vi "RRTAsynCall.vi"(8 "error in (no error)":errorcluster, 9 "appended path":path, 10 "VI Refnum":refnum<vi>, 11 "Input":T1={"seed"=500000, "pathsize"=0, "probGoal"=0.1, "probWaypoint"=0.6, "step"=10.0, "threshold"=10.0, "field_length"=9000.0, "field_width"=6000.0, "startAndEnd"=[[0.0, 0.0], [0.0, 0.0]], "obsList"=[[0.0, 0.0]], "obsLen"=1, "lastTree"=[[0.0, 0.0]], "lastTreeLen"=1, "newTree"=array[1012 elements], "useSimplePath"=0, "debug"=0.0}) -> (0 "error out":errorcluster, 3 "Output":T2)   [LabVIEW 2023]
uses:
  RRTOutput.ctl
  RRTInput.ctl
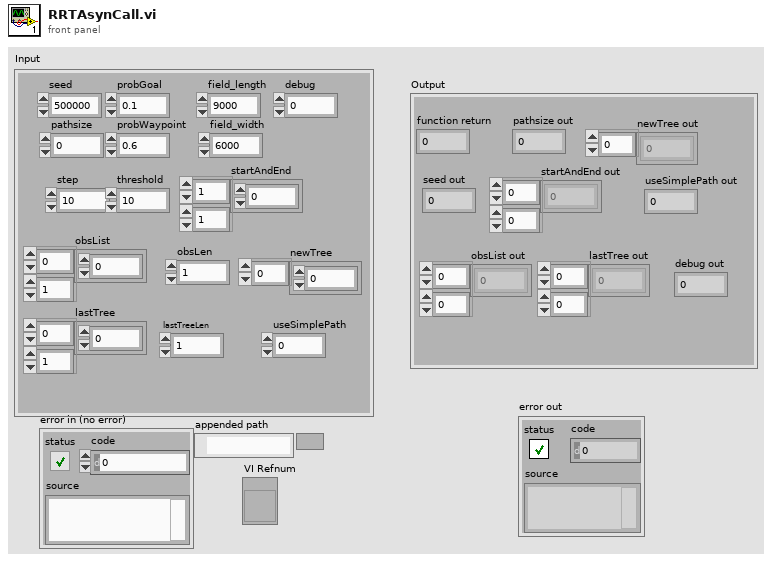
[diagram p1: front panel]
types:
  T1 = typedef "RRTInput.ctl" = cluster{"seed":i32, "pathsize":i32, "probGoal":sgl, "probWaypoint":sgl, "step":sgl, "threshold":sgl, "field_length":sgl, "field_width":sgl, "startAndEnd":sgl[][], "obsList":sgl[][], "obsLen":i32, "lastTree":sgl[][], "lastTreeLen":i32, "newTree":sgl[], "useSimplePath":i32, "debug":sgl}
  T2 = typedef "RRTOutput.ctl" = cluster{"function return":i32, "seed out":i32, "pathsize out":i32, "startAndEnd out":sgl[][], "obsList out":sgl[][], "lastTree out":sgl[][], "newTree out":sgl[], "useSimplePath out":i32, "debug out":sgl}
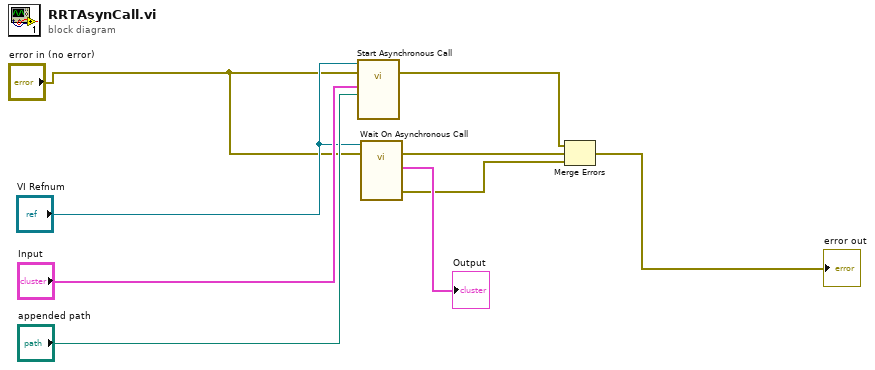
[diagram p0: block diagram]
diagram:
  n1 = call-by-ref "Start Asynchronous Call"(reference="VI Refnum", error in="error in (no error)", "DLL Path"="appended path", "Input"="Input") -> (error out=w4:errorcluster)  [unwired: 8 in, 3 out]
  n2 = call-by-ref "Wait On Asynchronous Call"(reference="VI Refnum", error in="error in (no error)") -> (error out=w3:errorcluster, 0:"error out"=w1:errorcluster, "Output"=→"Output":T2)  [unwired: 10 in, 1 out]
  n3 = Merge Errors(w4, w3, w1) -> (→"error out":errorcluster)
